vi "ATF Storage-AO Data.vi"(7 "Enum":enum16{"Write", "Read"}(ring), 11 "In_DO data":waveform(dbl)[](array[waveform])) -> (3 "out_DO data":waveform(dbl)[](array[waveform]))   [LabVIEW 2022 SP3]
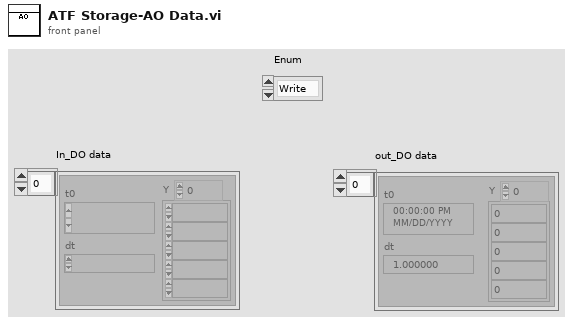
[diagram p1: front panel]
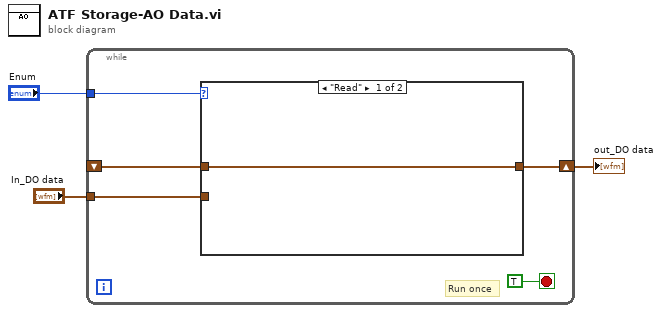
[diagram p0: block diagram]
diagram:
  n1 = while {
    tunnel: "Enum" -> [w7]
    tunnel: "In_DO data" -> [w6]
    shift-right: [w5] -> w3
    shift-left: _ -> [w4]
    stop <- TRUE stop-if-true
    # "Run once"
    n2 = case shown="\"Read\"" w7 {
      tunnel: w6 -> [_ w10]
      tunnel: [w9 w10] -> w5
      tunnel: w4 -> [w9 _]
      frame "Read" {
      }
      frame "Write" {
      }
    }
  }
  "out_DO data" <- w3
